vi "Screwed Up Periodic Tasks.vi"(8 "error in":errorcluster) -> ()   [LabVIEW 2014]
doc: "This VI runs in parallel to other tasks. It can contain as many user-defined periodic loops as you need. These can carry out PID or other sorts of timed response."
uses:
  <vilib>/Rock Robotics/WPI/Joystick/WPI_JoystickGetSetRefNum.vi
  <vilib>/Rock Robotics/WPI/RobotDrive/WPI_RobotDriveGetSetRefNum.vi
  Robot Global Data.vi
panel:
  in  "State":string
  out "Photoeye":bool
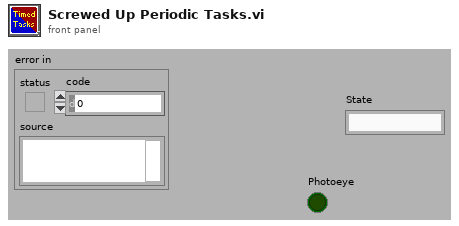
[diagram p1: front panel]
types:
  T1 = typedef "WPI_JoystickDevRef.ctl" = cluster{"Device":T2}
  T2 = typedef "WPI_JoystickDeviceEnum.ctl" = enum16{"USB 0", "USB 1", "USB 2", "USB 3", "USB 4", "USB 5"}
  T3 = typedef "WPI_RobotDriveDevRef.ctl" = cluster{"DevStatus":errorcluster, "Motors[]":T4[], "Square Inputs":bool, "Max Output":dbl}
  T4 = typedef "WPI_MotorControlDeviceRef.ctl" = cluster{"DeviceStatus":errorcluster, "Type":T5, "PWM":cluster{"Controller":T6, "PWM Channel":T7, "DeadBand":T8}, "CAN":cluster{"Device Number":u8, "Control Mode":T9, "Semaphore":T10, "Max Vout":dbl, "TalonSRX Control Mode":T11}, "Invert":bool, "TransformRef":T12, "InvTransformRef":T12}
  T5 = typedef "WPI_MotorControlType.ctl" = enum16{"PWM", "CAN", "CANTalonSRX"}
  T6 = typedef "FPGA_TypedefDigitalModule.ctl" = enum16{"Controller 1"}
  T7 = typedef "FPGA_DIOPWMChannel.ctl" = enum8{"PWM 0", "PWM 1", "PWM 2", "PWM 3", "PWM 4", "PWM 5", "PWM 6", "PWM 7", "PWM 8", "PWM 9", "PWM MXP 0", "PWM MXP 1", "PWM MXP 2", "PWM MXP 3", "PWM MXP 4", "PWM MXP 5", "PWM MXP 6", "PWM MXP 7", "PWM MXP 8", "PWM MXP 9", "Invalid"}
  T8 = typedef "WPI_PWMDeadband.ctl" = cluster{"Name":string, "maxPositivePwm":i32, "minPositivePwm":i32, "centerPwm":i32, "maxNegativePwm":i32, "minNegativePwm":i32, "angularRange":u16}
  T9 = typedef "WPI_CANJaguar_ControlMode.ctl" = enum8{"Percent VBus", "Current", "Speed", "Position", "Voltage"}
  T10 = typedef "Semaphore RefNum" = refnum<k1>
  T11 = typedef "WPI_CANTalonSRX_APIControlMode.ctl" = enum8{"Percent VBus", "Speed", "Position", "Slave", "Unchanged / Invalid"}
  T12 = typedef "WPI_PWMTransform_ConPane.ctl" = refnum<vi>
  T13 = cluster{"JoystickDevRef":T1, "RobotDriveDevRef":T3}
  T14 = typedef "WPI_ServoDeviceRef.ctl" = cluster{"DeviceStatus":errorcluster, "Controller":T6, "PWM Channel":T7, "DeadBand":T8}
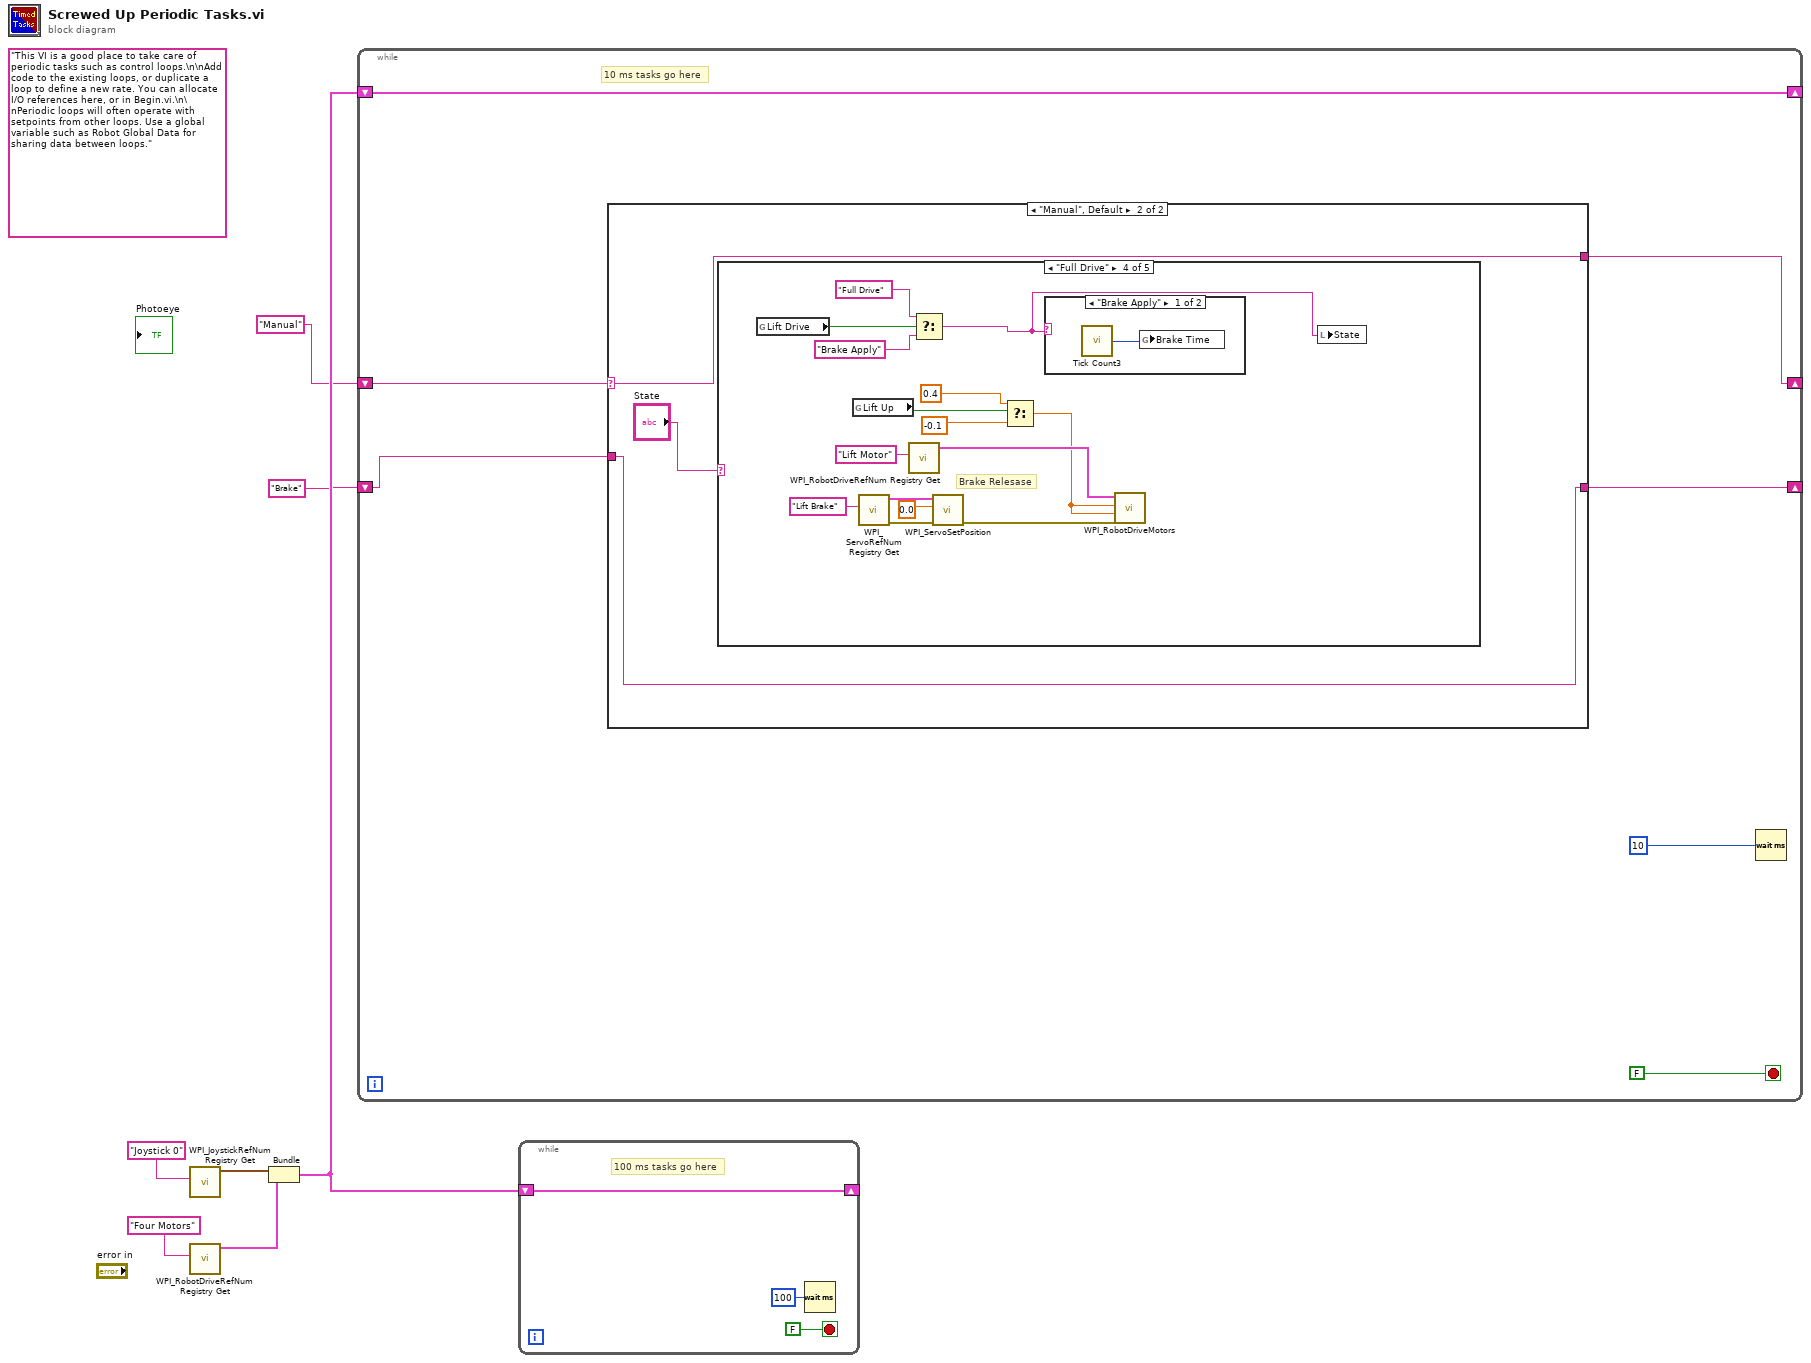
[diagram p0: block diagram]
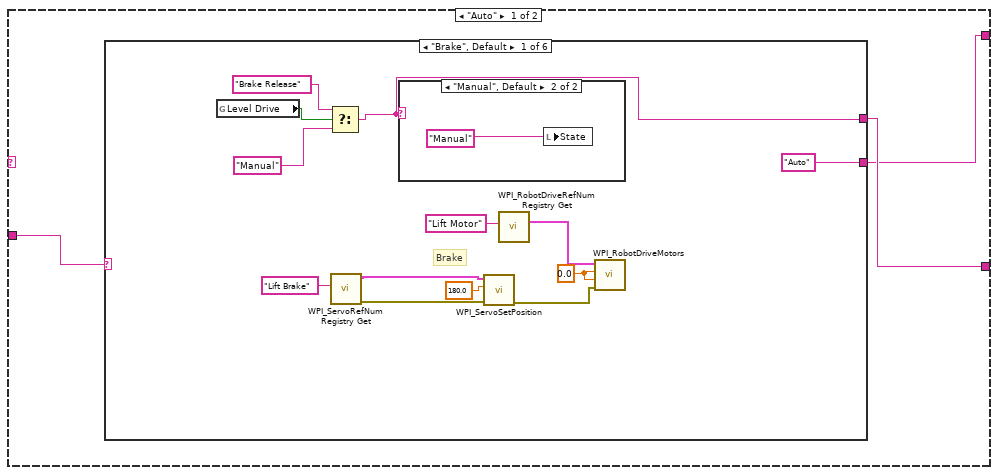
[diagram p2: hidden frame]
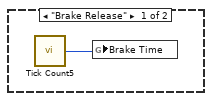
[diagram p3: hidden frame]
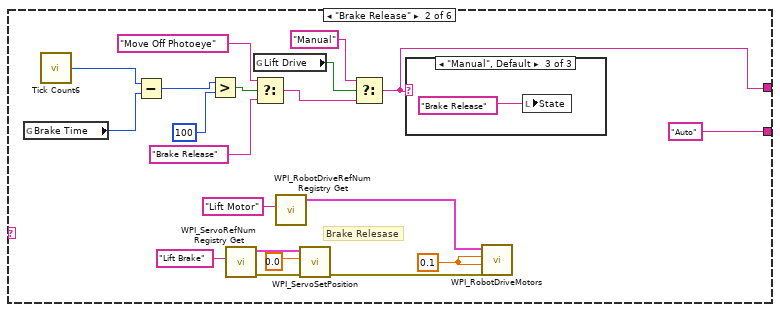
[diagram p4: hidden frame]
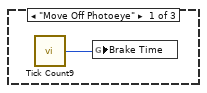
[diagram p5: hidden frame]
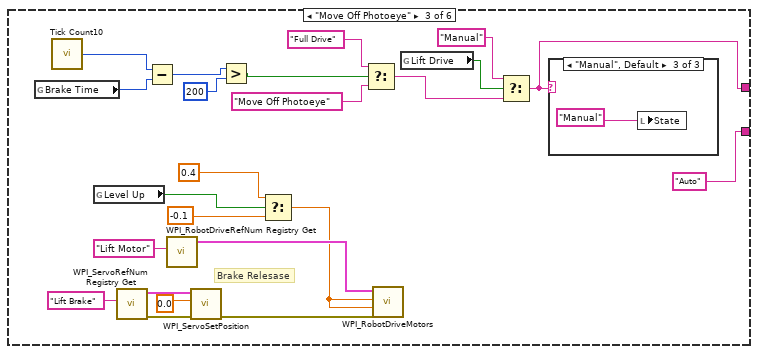
[diagram p7: hidden frame]
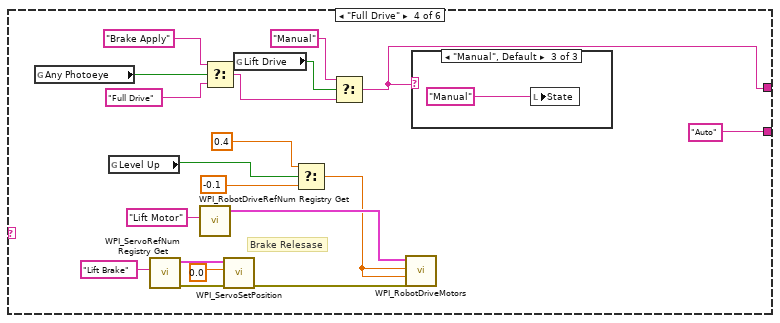
[diagram p10: hidden frame]
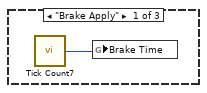
[diagram p11: hidden frame]
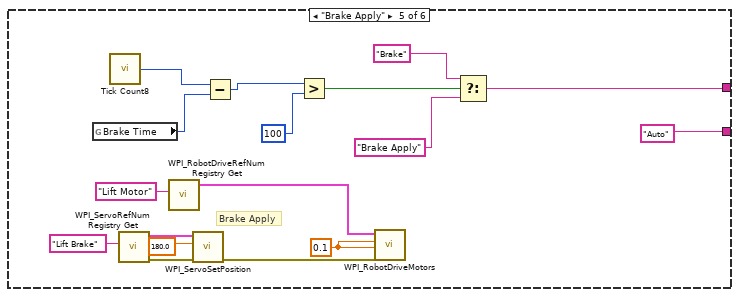
[diagram p13: hidden frame]
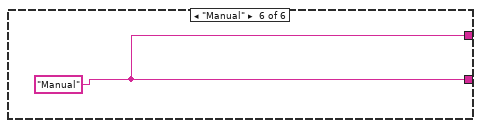
[diagram p14: hidden frame]
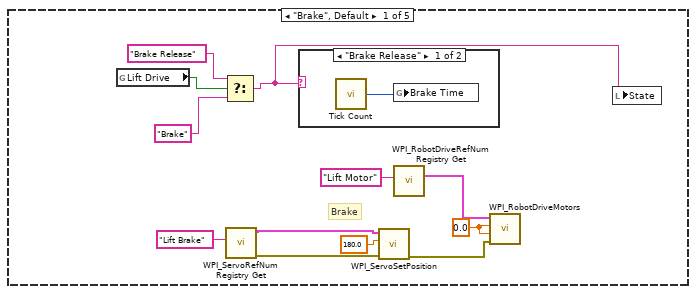
[diagram p15: hidden frame]
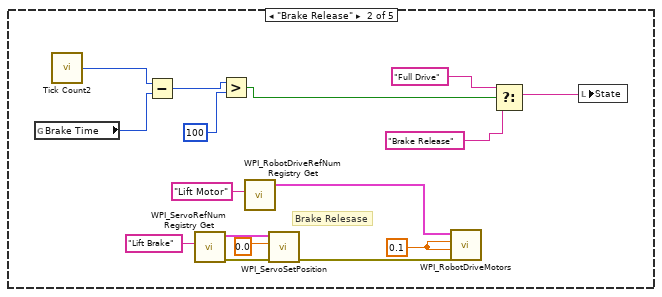
[diagram p17: hidden frame]
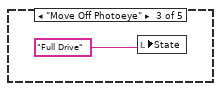
[diagram p18: hidden frame]
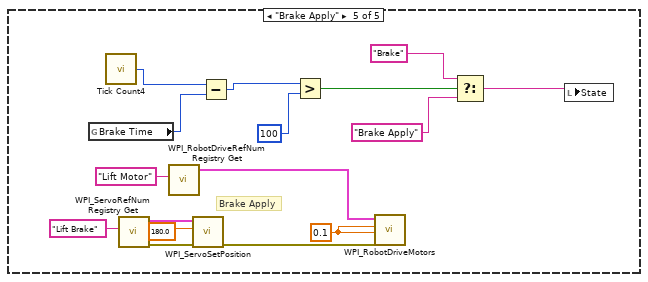
[diagram p20: hidden frame]
diagram:
  (unwired) "This VI is a good place to take care of periodic tasks such as control loops.\n\nAdd code to the existing loops, or duplicate a loop to define a new rate. You can allocate I/O references here, or in Begin.vi.\n\nPeriodic loops will often operate with setpoints from other loops. Use a global variable such as Robot Global Data for sharing data between loops."
  n1 = call <vilib>:"WPI_JoystickRefNum Registry Get.vi"("refnum name"="Joystick 0") -> ("JoystickDevRef"=w5:T1)  [unwired: 1 in, 9 out]
  n2 = call <vilib>:"WPI_RobotDriveRefNum Registry Get.vi"("refnum name"="Four Motors") -> ("RobotDriveDevRef"=w4:T3)  [unwired: 1 in, 9 out]
  n3 = Bundle("JoystickDevRef"=w5, "RobotDriveDevRef"=w4) -> (w3:T13)  [unwired: 1 out]
  n4 = while {
    shift-right: [w12] -> _
    shift-left: w3 -> [w12]
    shift-right: [w10] -> _
    shift-left: "Brake" -> [w11]
    shift-right: [w8] -> _
    shift-left: "Manual" -> [w9]
    stop <- FALSE stop-if-true
    # "10 ms tasks go here"
    n5 = case shown="\"Manual\", Default" w9 {
      selector: w9 -> [_ w119]
      tunnel: w11 -> [w17 w118]
      tunnel: [w16 w118] -> w10
      tunnel: [w15 w119] -> w8
      frame "Auto" {
        n6 = case shown="\"Brake\", Default" w17 {
          tunnel: [w19 w36 w56 w80 w106 w117] -> w16
          tunnel: ["Auto" "Auto" "Auto" "Auto" "Auto" w117] -> w15
          frame "Brake", Default {
            w25 = 0.0 ("LeftSpeed")
            # "Brake"
            n7 = global read "Robot Global Data.vi" "Level Drive"() -> (w22:bool)
            n8 = Select(t="Brake Release", s=w22, f="Manual") -> (s? t:f=w19:string)
            n9 = call <vilib>:"WPI_ServoRefNum Registry Get.vi"("refnum name"="Lift Brake") -> ("error out"=w23:errorcluster, "ServoDeviceRef"=w28:T14)  [unwired: 9 in]
            n10 = case shown="\"Manual\", Default" w19 {
              frame "Brake Release" {
                n11 = call "Tick Count5"() -> ("Tick Count(mSec)"=w31:u32)
                n12 = global write "Robot Global Data.vi" "Brake Time"(w31) -> ()
              }
              frame "Manual", Default {
                n13 = local write "State"("Manual" ("t")) -> ()
              }
            }
            n14 = call <vilib>:"WPI_ServoSetPosition.vi"("error in (no error)"=w23, "Position"=180.0, "ServoDeviceRef"=w28) -> ("error out"=w24:errorcluster)  [unwired: 7 in, 1 out]
            n15 = call <vilib>:"WPI_RobotDriveRefNum Registry Get.vi"("refnum name"="Lift Motor") -> ("RobotDriveDevRef"=w26:T3)  [unwired: 9 in, 1 out]
            n16 = call <vilib>:"WPI_RobotDriveMotors.vi"("error in (no error)"=w24, "RightSpeed"=w25, "LeftSpeed"=w25, "RobotDriveDevRef"=w26) -> ()  [unwired: 5 in, 3 out]
          }
          frame "Brake Release" {
            w45 = 0.1 ("RightSpeed")
            # "Brake Relesase"
            n17 = global read "Robot Global Data.vi" "Brake Time"() -> (w38:u32)
            n18 = call "Tick Count6"() -> ("Tick Count(mSec)"=w39:u32)
            n19 = Subtract(x=w39, y=w38) -> (x-y=w42:u32)
            n20 = Greater?(x=w42, y=u32 100) -> (0:w43:bool)
            n21 = call <vilib>:"WPI_ServoRefNum Registry Get.vi"("refnum name"="Lift Brake") -> ("error out"=w47:errorcluster, "ServoDeviceRef"=w50:T14)  [unwired: 9 in]
            n22 = global read "Robot Global Data.vi" "Lift Drive"() -> (w35:bool)
            n23 = Select(t="Move Off Photoeye", s=w43, f="Brake Release") -> (s? t:f=w37:string)
            n24 = call <vilib>:"WPI_RobotDriveRefNum Registry Get.vi"("refnum name"="Lift Motor") -> ("RobotDriveDevRef"=w48:T3)  [unwired: 9 in, 1 out]
            n25 = call <vilib>:"WPI_ServoSetPosition.vi"("error in (no error)"=w47, "Position"=0.0, "ServoDeviceRef"=w50) -> ("error out"=w46:errorcluster)  [unwired: 7 in, 1 out]
            n26 = Select(t="Manual", s=w35, f=w37) -> (s? t:f=w36:string)
            n27 = case shown="\"Manual\", Default" w36 {
              frame "Move Off Photoeye" {
                n28 = call "Tick Count9"() -> ("Tick Count(mSec)"=w53:u32)
                n29 = global write "Robot Global Data.vi" "Brake Time"(w53) -> ()
              }
              frame "Break Release" {
              }
              frame "Manual", Default {
                n30 = local write "State"("Brake Release") -> ()
              }
            }
            n31 = call <vilib>:"WPI_RobotDriveMotors.vi"("error in (no error)"=w46, "RightSpeed"=w45, "LeftSpeed"=w45, "RobotDriveDevRef"=w48) -> ()  [unwired: 5 in, 3 out]
          }
          frame "Move Off Photoeye" {
            # "Brake Relesase"
            n32 = global read "Robot Global Data.vi" "Brake Time"() -> (w61:u32)
            n33 = call "Tick Count10"() -> ("Tick Count(mSec)"=w62:u32)
            n34 = global read "Robot Global Data.vi" "Level Up"() -> (w68:bool)
            n35 = call <vilib>:"WPI_ServoRefNum Registry Get.vi"("refnum name"="Lift Brake") -> ("error out"=w72:errorcluster, "ServoDeviceRef"=w75:T14)  [unwired: 9 in]
            n36 = Subtract(x=w62, y=w61) -> (x-y=w64:u32)
            n37 = call <vilib>:"WPI_RobotDriveRefNum Registry Get.vi"("refnum name"="Lift Motor") -> ("RobotDriveDevRef"=w73:T3)  [unwired: 9 in, 1 out]
            n38 = call <vilib>:"WPI_ServoSetPosition.vi"("error in (no error)"=w72, "Position"=0.0, "ServoDeviceRef"=w75) -> ("error out"=w71:errorcluster)  [unwired: 7 in, 1 out]
            n39 = Greater?(x=w64, y=u32 200) -> (0:w60:bool)
            n40 = Select(t=0.4 ("RightSpeed"), s=w68, f=-0.1) -> (s? t:f=w70:dbl)
            n41 = Select(t="Full Drive", s=w60, f="Move Off Photoeye") -> (s? t:f=w57:string)
            n42 = call <vilib>:"WPI_RobotDriveMotors.vi"("error in (no error)"=w71, "RightSpeed"=w70, "LeftSpeed"=w70, "RobotDriveDevRef"=w73) -> ()  [unwired: 5 in, 3 out]
            n43 = global read "Robot Global Data.vi" "Lift Drive"() -> (w59:bool)
            n44 = Select(t="Manual", s=w59, f=w57) -> (s? t:f=w56:string)
            n45 = case shown="\"Manual\", Default" w56 {
              frame "Move Off Photoeye" {
              }
              frame "Full Drive" {
              }
              frame "Manual", Default {
                n46 = local write "State"("Manual" ("t")) -> ()
              }
            }
          }
          frame "Full Drive" {
            # "Brake Relesase"
            n47 = global read "Robot Global Data.vi" "Any Photoeye"() -> (w87:bool)
            n48 = global read "Robot Global Data.vi" "Level Up"() -> (w88:bool)
            n49 = call <vilib>:"WPI_ServoRefNum Registry Get.vi"("refnum name"="Lift Brake") -> ("error out"=w92:errorcluster, "ServoDeviceRef"=w95:T14)  [unwired: 9 in]
            n50 = call <vilib>:"WPI_RobotDriveRefNum Registry Get.vi"("refnum name"="Lift Motor") -> ("RobotDriveDevRef"=w93:T3)  [unwired: 9 in, 1 out]
            n51 = Select(t="Brake Apply", s=w87, f="Full Drive") -> (s? t:f=w81:string)
            n52 = call <vilib>:"WPI_ServoSetPosition.vi"("error in (no error)"=w92, "Position"=0.0, "ServoDeviceRef"=w95) -> ("error out"=w91:errorcluster)  [unwired: 7 in, 1 out]
            n53 = global read "Robot Global Data.vi" "Lift Drive"() -> (w83:bool)
            n54 = Select(t=0.4 ("RightSpeed"), s=w88, f=-0.1) -> (s? t:f=w90:dbl)
            n55 = Select(t="Manual", s=w83, f=w81) -> (s? t:f=w80:string)
            n56 = call <vilib>:"WPI_RobotDriveMotors.vi"("error in (no error)"=w91, "RightSpeed"=w90, "LeftSpeed"=w90, "RobotDriveDevRef"=w93) -> ()  [unwired: 5 in, 3 out]
            n57 = case shown="\"Manual\", Default" w80 {
              frame "Brake Apply" {
                n58 = call "Tick Count7"() -> ("Tick Count(mSec)"=w98:u32)
                n59 = global write "Robot Global Data.vi" "Brake Time"(w98) -> ()
              }
              frame "Full Drive" {
              }
              frame "Manual", Default {
                n60 = local write "State"("Manual" ("t")) -> ()
              }
            }
          }
          frame "Brake Apply" {
            w116 = 0.1 ("RightSpeed")
            # "Brake Apply"
            n61 = global read "Robot Global Data.vi" "Brake Time"() -> (w102:u32)
            n62 = call "Tick Count8"() -> ("Tick Count(mSec)"=w103:u32)
            n63 = call <vilib>:"WPI_ServoRefNum Registry Get.vi"("refnum name"="Lift Brake") -> ("error out"=w114:errorcluster, "ServoDeviceRef"=w111:T14)  [unwired: 9 in]
            n64 = call <vilib>:"WPI_RobotDriveRefNum Registry Get.vi"("refnum name"="Lift Motor") -> ("RobotDriveDevRef"=w113:T3)  [unwired: 9 in, 1 out]
            n65 = call <vilib>:"WPI_ServoSetPosition.vi"("error in (no error)"=w114, "Position"=180.0, "ServoDeviceRef"=w111) -> ("error out"=w115:errorcluster)  [unwired: 7 in, 1 out]
            n66 = Subtract(x=w103, y=w102) -> (x-y=w101:u32)
            n67 = Greater?(x=w101, y=u32 100) -> (0:w104:bool)
            n68 = call <vilib>:"WPI_RobotDriveMotors.vi"("error in (no error)"=w115, "RightSpeed"=w116, "LeftSpeed"=w116, "RobotDriveDevRef"=w113) -> ()  [unwired: 5 in, 3 out]
            n69 = Select(t="Brake", s=w104, f="Brake Apply") -> (s? t:f=w106:string)
          }
          frame "Manual" {
            w117 = "Manual"
          }
        }
      }
      frame "Manual", Default {
        n70 = case shown="\"Full Drive\"" "State" {
          frame "Brake", Default {
            w127 = 0.0 ("LeftSpeed")
            # "Brake"
            n71 = global read "Robot Global Data.vi" "Lift Drive"() -> (w124:bool)
            n72 = Select(t="Brake Release", s=w124, f="Brake") -> (s? t:f=w121:string)
            n73 = call <vilib>:"WPI_ServoRefNum Registry Get.vi"("refnum name"="Lift Brake") -> ("error out"=w125:errorcluster, "ServoDeviceRef"=w130:T14)  [unwired: 9 in]
            n74 = case shown="\"Brake Release\"" w121 {
              frame "Brake Release" {
                n75 = call "Tick Count"() -> ("Tick Count(mSec)"=w133:u32)
                n76 = global write "Robot Global Data.vi" "Brake Time"(w133) -> ()
              }
              frame "Brake", Default {
              }
            }
            n77 = call <vilib>:"WPI_ServoSetPosition.vi"("error in (no error)"=w125, "Position"=180.0, "ServoDeviceRef"=w130) -> ("error out"=w126:errorcluster)  [unwired: 7 in, 1 out]
            n78 = call <vilib>:"WPI_RobotDriveRefNum Registry Get.vi"("refnum name"="Lift Motor") -> ("RobotDriveDevRef"=w128:T3)  [unwired: 9 in, 1 out]
            n79 = call <vilib>:"WPI_RobotDriveMotors.vi"("error in (no error)"=w126, "RightSpeed"=w127, "LeftSpeed"=w127, "RobotDriveDevRef"=w128) -> ()  [unwired: 5 in, 3 out]
            n80 = local write "State"(w121) -> ()
          }
          frame "Brake Release" {
            w142 = 0.1 ("RightSpeed")
            # "Brake Relesase"
            n81 = global read "Robot Global Data.vi" "Brake Time"() -> (w135:u32)
            n82 = call "Tick Count2"() -> ("Tick Count(mSec)"=w136:u32)
            n83 = Subtract(x=w136, y=w135) -> (x-y=w139:u32)
            n84 = call <vilib>:"WPI_ServoRefNum Registry Get.vi"("refnum name"="Lift Brake") -> ("error out"=w144:errorcluster, "ServoDeviceRef"=w147:T14)  [unwired: 9 in]
            n85 = Greater?(x=w139, y=u32 100) -> (0:w140:bool)
            n86 = call <vilib>:"WPI_RobotDriveRefNum Registry Get.vi"("refnum name"="Lift Motor") -> ("RobotDriveDevRef"=w145:T3)  [unwired: 9 in, 1 out]
            n87 = call <vilib>:"WPI_ServoSetPosition.vi"("error in (no error)"=w144, "Position"=0.0, "ServoDeviceRef"=w147) -> ("error out"=w143:errorcluster)  [unwired: 7 in, 1 out]
            n88 = call <vilib>:"WPI_RobotDriveMotors.vi"("error in (no error)"=w143, "RightSpeed"=w142, "LeftSpeed"=w142, "RobotDriveDevRef"=w145) -> ()  [unwired: 5 in, 3 out]
            n89 = Select(t="Full Drive", s=w140, f="Brake Release") -> (s? t:f=w134:string)
            n90 = local write "State"(w134) -> ()
          }
          frame "Move Off Photoeye" {
            n91 = local write "State"("Full Drive" ("t")) -> ()
          }
          frame "Full Drive" {
            # "Brake Relesase"
            n92 = global read "Robot Global Data.vi" "Lift Drive"() -> (w155:bool)
            n93 = global read "Robot Global Data.vi" "Lift Up"() -> (w156:bool)
            n94 = call <vilib>:"WPI_ServoRefNum Registry Get.vi"("refnum name"="Lift Brake") -> ("error out"=w160:errorcluster, "ServoDeviceRef"=w163:T14)  [unwired: 9 in]
            n95 = call <vilib>:"WPI_RobotDriveRefNum Registry Get.vi"("refnum name"="Lift Motor") -> ("RobotDriveDevRef"=w161:T3)  [unwired: 9 in, 1 out]
            n96 = Select(t="Full Drive", s=w155, f="Brake Apply") -> (s? t:f=w151:string)
            n97 = call <vilib>:"WPI_ServoSetPosition.vi"("error in (no error)"=w160, "Position"=0.0, "ServoDeviceRef"=w163) -> ("error out"=w159:errorcluster)  [unwired: 7 in, 1 out]
            n98 = Select(t=0.4 ("RightSpeed"), s=w156, f=-0.1) -> (s? t:f=w158:dbl)
            n99 = case shown="\"Brake Apply\"" w151 {
              frame "Brake Apply" {
                n100 = call "Tick Count3"() -> ("Tick Count(mSec)"=w166:u32)
                n101 = global write "Robot Global Data.vi" "Brake Time"(w166) -> ()
              }
              frame "Full Drive", Default {
              }
            }
            n102 = call <vilib>:"WPI_RobotDriveMotors.vi"("error in (no error)"=w159, "RightSpeed"=w158, "LeftSpeed"=w158, "RobotDriveDevRef"=w161) -> ()  [unwired: 5 in, 3 out]
            n103 = local write "State"(w151) -> ()
          }
          frame "Brake Apply" {
            w182 = 0.1 ("RightSpeed")
            # "Brake Apply"
            n104 = global read "Robot Global Data.vi" "Brake Time"() -> (w169:u32)
            n105 = call "Tick Count4"() -> ("Tick Count(mSec)"=w170:u32)
            n106 = call <vilib>:"WPI_ServoRefNum Registry Get.vi"("refnum name"="Lift Brake") -> ("error out"=w180:errorcluster, "ServoDeviceRef"=w177:T14)  [unwired: 9 in]
            n107 = call <vilib>:"WPI_RobotDriveRefNum Registry Get.vi"("refnum name"="Lift Motor") -> ("RobotDriveDevRef"=w179:T3)  [unwired: 9 in, 1 out]
            n108 = call <vilib>:"WPI_ServoSetPosition.vi"("error in (no error)"=w180, "Position"=180.0, "ServoDeviceRef"=w177) -> ("error out"=w181:errorcluster)  [unwired: 7 in, 1 out]
            n109 = Subtract(x=w170, y=w169) -> (x-y=w168:u32)
            n110 = Greater?(x=w168, y=u32 100) -> (0:w171:bool)
            n111 = call <vilib>:"WPI_RobotDriveMotors.vi"("error in (no error)"=w181, "RightSpeed"=w182, "LeftSpeed"=w182, "RobotDriveDevRef"=w179) -> ()  [unwired: 5 in, 3 out]
            n112 = Select(t="Brake", s=w171, f="Brake Apply") -> (s? t:f=w167:string)
            n113 = local write "State"(w167) -> ()
          }
        }
      }
    }
    n114 = Wait (ms)(milliseconds to wait=u32 10) -> ()  [unwired: 1 out]
  }
  n115 = while {
    shift-right: [w183] -> _
    shift-left: w3 -> [w183]
    stop <- FALSE stop-if-true
    # "100 ms tasks go here"
    n116 = Wait (ms)(milliseconds to wait=u32 100) -> ()  [unwired: 1 out]
  }
